vi "Wait.vi"(7 "Reference in":T1={"Device"="", "Function"="", "delay"=20}, 8 "error in (no error)":errorcluster, 11 "Device in":refnum<visa-resource-name>) -> (0 "error out":errorcluster, 3 "Device out":refnum<visa-resource-name>)   [LabVIEW 2021, in "Rigol DM3052.lvlib"]
uses:
  Rigol DM3052.lvlib
  Reference.ctl
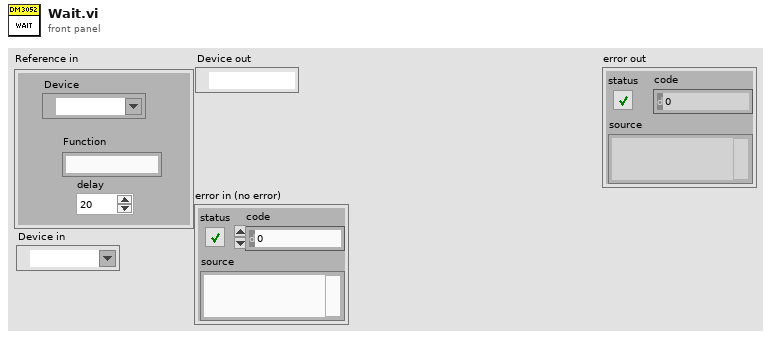
[diagram p1: front panel]
types:
  T1 = typedef "Rigol DM3052.lvlib/Reference.ctl" = cluster{"Device":refnum<visa-resource-name>, "Function":string, "delay":u32}
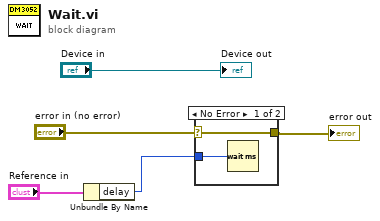
[diagram p0: block diagram]
diagram:
  n1 = Unbundle By Name("Reference in") -> ("delay"=w4:u32)
  n2 = case shown="No Error" "error in (no error)" {
    selector: "error in (no error)" -> [w7 w8]
    tunnel: [w7 w8] -> w2
    tunnel: w4 -> [w6 _]
    frame No Error {
      n3 = Wait (ms)(milliseconds to wait=w6) -> ()  [unwired: 1 out]
    }
    frame Error {
    }
  }
  "error out" <- w2
  "Device out" <- "Device in"
